vi "AlloysLogger.vi"() -> ()   [LabVIEW 2014]
uses:
  Typedef_FindPortActions.ctl
  Typedef_TeachLabArduinos.ctl
  Typedef_DataLogger_Actions.ctl
  <vilib>/Utility/file.llb/Write To Spreadsheet File (DBL).vi
panel:
  in  "Time Step (ms)":i32=100 min=5 max=5000 step=1
  out "Elapsed Time (s)":dbl format="%.1f"
  out "Temperature (°C)":dbl format="%.1f"
  in  "Filename Header":string="Data"
  in  "Maximum Log Time (s)":dbl=3600.0
  out "Status":enum16{"Logging", "Stopped"}(ring)=enum."Stopped"
  in  "Logging":cluster{"Start":bool, "Stop":bool}
  out "Last Save's Filename":string
  in  "Save Data":bool
  in  "Reset Graph":bool
  out "XY Graph":cluster{dbl[], dbl[]}(graph)
  out "Error Out":errorcluster
  in  "Exit Program":bool
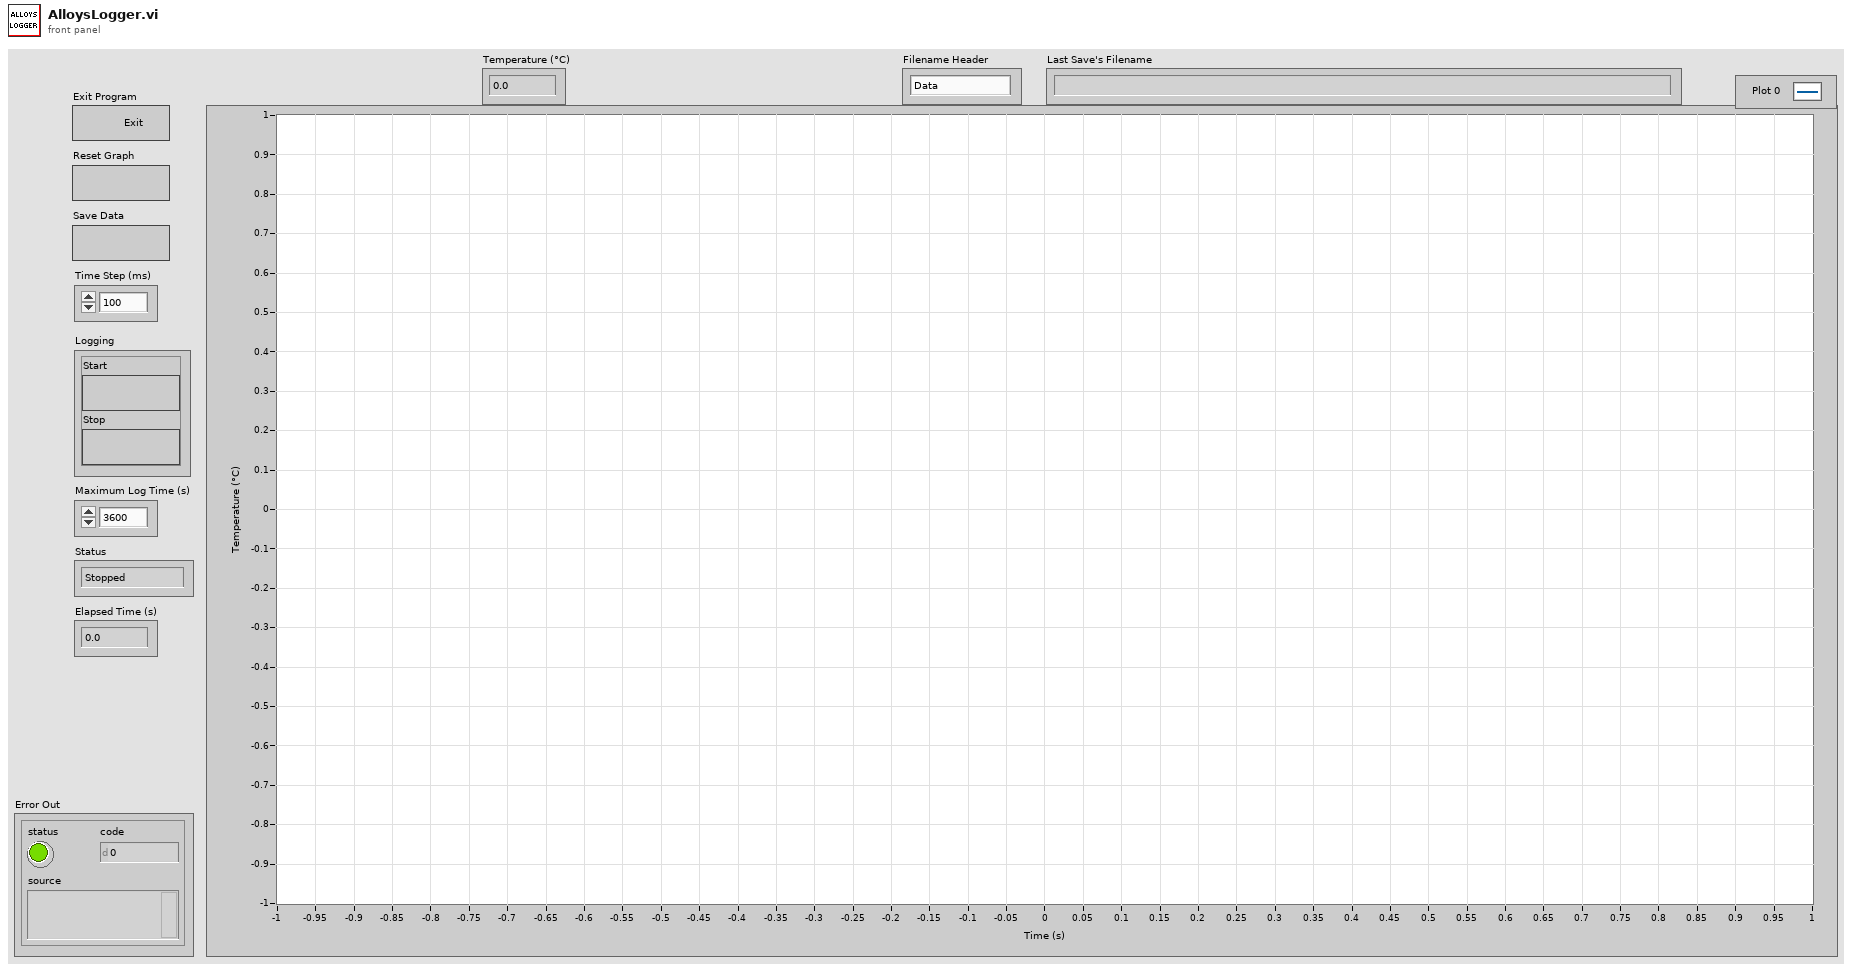
[diagram p1: front panel]
types:
  T1 = typedef "Typedef_FindPortActions.ctl" = enum16{"Reset List", "Find arduinos", "Get COM Port"}
  T2 = typedef "Typedef_TeachLabArduinos.ctl" = enum16{"FH", "AL", "CO"}
  T3 = typedef "Typedef_DataLogger_Actions.ctl" = enum16{"Connect", "Disconnect", "Get Reading", "Set Offset", "Get Offset", "Set Time Step", "Get Time Step", "Save Settings", "Disable Readings", "Enable Readings"}
  T4 = enum32{"invalid app kind", "Development System", "Run Time System", "Student Edition", "Embedded LabVIEW", "Evaluation", "Custom"}
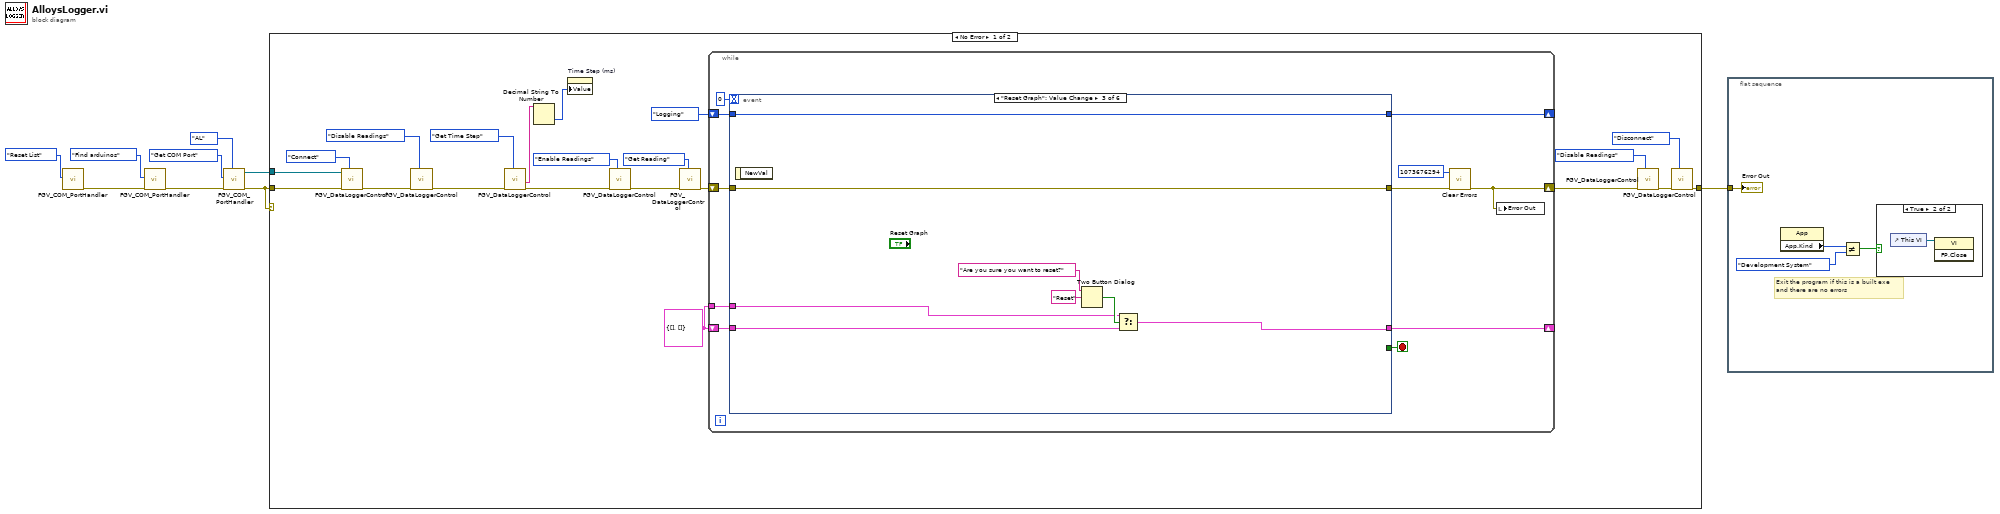
[diagram p0: block diagram]
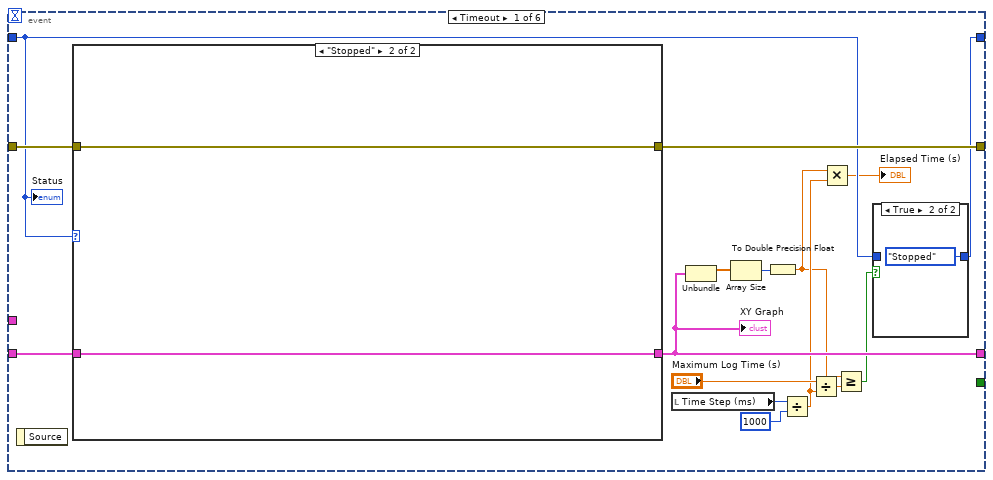
[diagram p3: hidden frame]
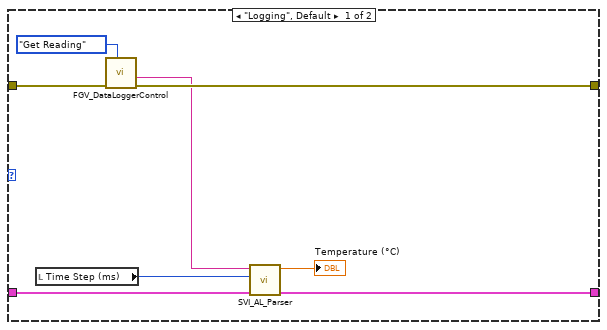
[diagram p5: hidden frame]
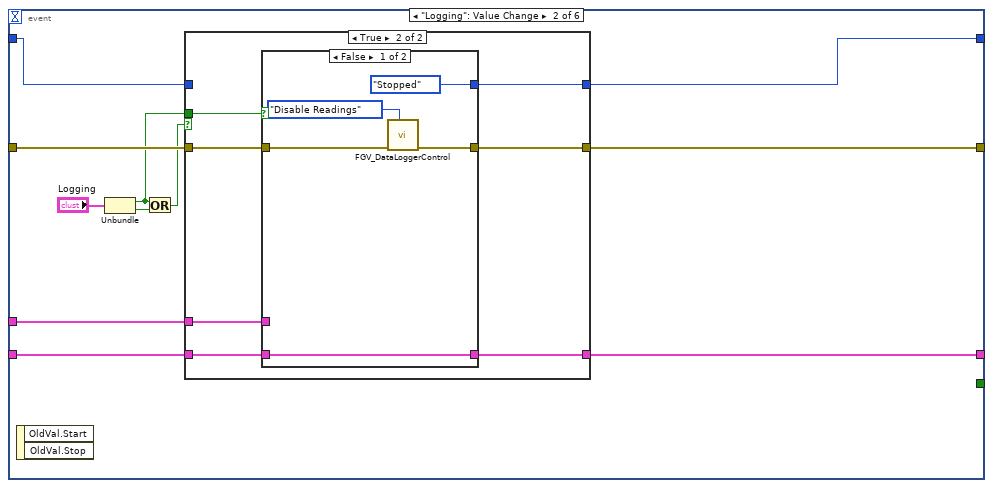
[diagram p6: hidden frame]
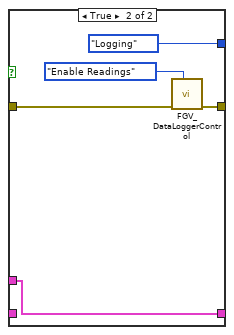
[diagram p8: hidden frame]
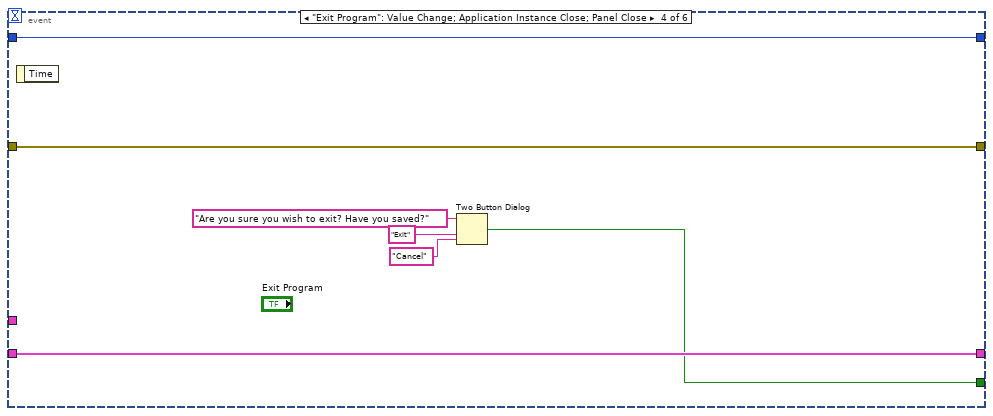
[diagram p9: hidden frame]
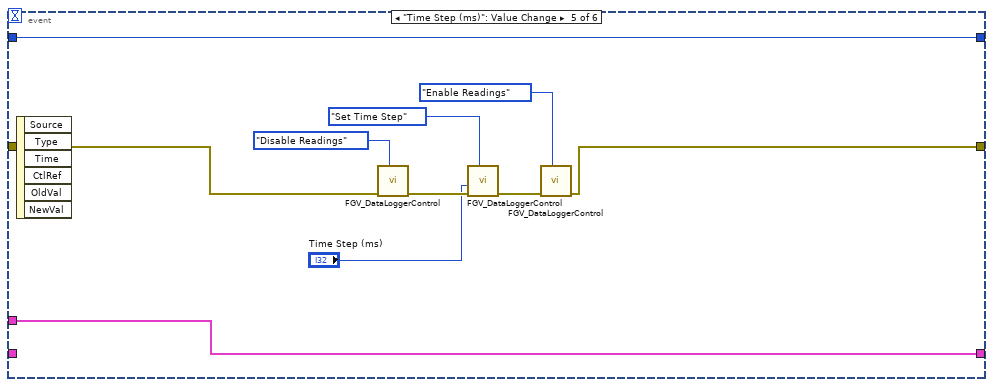
[diagram p10: hidden frame]
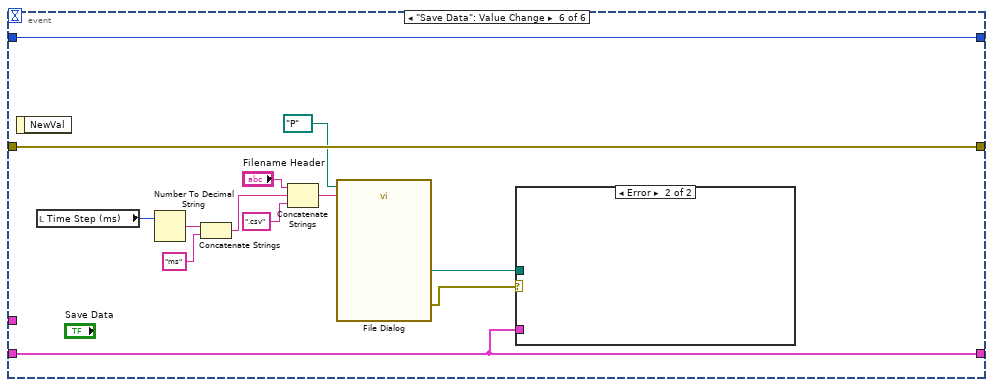
[diagram p11: hidden frame]
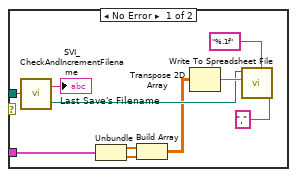
[diagram p12: hidden frame]
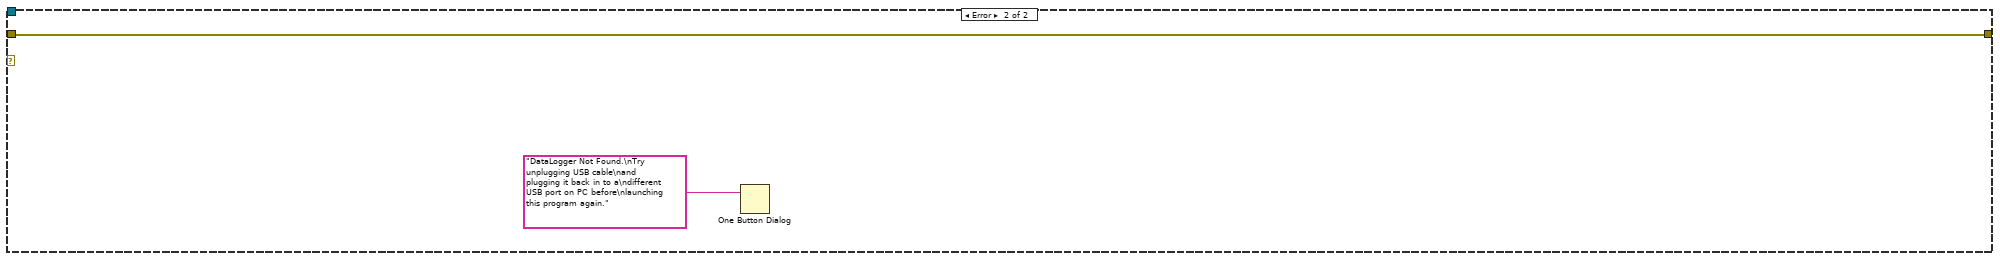
[diagram p13: hidden frame]
diagram:
  n1 = call "FGV_COM_PortHandler.vi"("Action"=Typedef_FindPortActions."Reset List") -> ("Error Out"=w5:errorcluster)  [unwired: 5 in, 2 out]
  n2 = call "FGV_COM_PortHandler.vi"("Error In"=w5, "Action"=Typedef_FindPortActions."Find arduinos") -> ("Error Out"=w9:errorcluster)  [unwired: 4 in, 2 out]
  n3 = call "FGV_COM_PortHandler.vi"("Device"=Typedef_TeachLabArduinos."AL", "Error In"=w9, "Action"=Typedef_FindPortActions."Get COM Port") -> ("Error Out"=w1:errorcluster, "COM Port"=w3:refnum<visa-resource-name>)  [unwired: 3 in, 1 out]
  n4 = case shown="No Error" w1 {
    tunnel: w1 -> [w29 w150]
    tunnel: w3 -> [w28 _]
    tunnel: [w25 w150] -> w2
    frame No Error {
      w14 = cluster{dbl[], dbl[]} {[], []}
      n5 = call "FGV_DataLoggerControl.vi"("Actions"=Typedef_DataLogger_Actions."Connect", "Error In"=w29, "VISA Refnum in"=w28) -> ("Error Out"=w21:errorcluster)  [unwired: 6 in, 2 out]
      n6 = call "FGV_DataLoggerControl.vi"("Actions"=Typedef_DataLogger_Actions."Disable Readings", "Error In"=w21) -> ("Error Out"=w20:errorcluster)  [unwired: 7 in, 2 out]
      n7 = call "FGV_DataLoggerControl.vi"("Actions"=Typedef_DataLogger_Actions."Get Time Step", "Error In"=w20) -> ("Error Out"=w18:errorcluster, "read buffer"=w24:string)  [unwired: 7 in, 1 out]
      n8 = Decimal String To Number(string=w24) -> (number=w23:i32)  [unwired: 2 in, 1 out]
      n9 = property on="Time Step (ms)" class="DigNum (strict)"("Value"=w23) -> ()  [unwired: 2 in, 2 out]
      n10 = call "FGV_DataLoggerControl.vi"("Actions"=Typedef_DataLogger_Actions."Enable Readings", "Error In"=w18) -> ("Error Out"=w10:errorcluster)  [unwired: 7 in, 2 out]
      n11 = call "FGV_DataLoggerControl.vi"("Actions"=Typedef_DataLogger_Actions."Get Reading", "Error In"=w10) -> ("Error Out"=w11:errorcluster)  [unwired: 7 in, 2 out]
      n12 = while {
        shift-right: [w38] -> _
        shift-left: w14 -> [w37]
        tunnel: w14 -> [w36]
        shift-right: [w34] -> _
        shift-left: enum16{"Logging", "Stopped"}."Logging" ("Status") -> [w35]
        shift-right: [w32] -> w16
        shift-left: w11 -> [w41]
        stop <- w40 stop-if-true
        n13 = event shown="[2] \"Reset Graph\": Value Change" {
          selector: _ -> [_ _ _ _ _ _]
          dyn-events: _ -> [_ _ _ _ _ _]
          timeout: 0 -> [_ _ _ _ _ _]
          tunnel: w41 -> [w57 w78 w108 w114 w119 w138]
          tunnel: [w56 w77 w108 w114 w120 w138] -> w31
          tunnel: [_ _ _ w110 _ _] -> w40
          tunnel: [w53 w71 w101 w115 w118 w126] -> w38
          tunnel: w37 -> [w55 w72 w102 w115 _ w126]
          tunnel: w36 -> [_ w70 w103 _ w118 _]
          tunnel: [w46 w80 w107 w109 w117 w130] -> w34
          tunnel: w35 -> [w45 w79 w107 w109 w117 w130]
          event Timeout {
            n14 = event-data() -> ()  [unwired: 1 in, 1 out]
            n15 = case shown="\"Stopped\"" w45 {
              tunnel: w57 -> [w67 w68]
              tunnel: [w66 w68] -> w56
              tunnel: [w63 w69] -> w53
              tunnel: w55 -> [w62 w69]
              frame "Logging", Default {
                n16 = local read "Time Step (ms)"() -> (w60:i32)
                n17 = call "FGV_DataLoggerControl.vi"("Actions"=Typedef_DataLogger_Actions."Get Reading", "Error In"=w67) -> ("Error Out"=w66:errorcluster, "read buffer"=w64:string)  [unwired: 7 in, 1 out]
                n18 = call "SVI_AL_Parser.vi"("Cluster in"=w62, "Time Step (ms)"=w60, "read buffer"=w64) -> ("Cluster out"=w63:cluster{"Array":dbl[], "Array":dbl[]}, "Temperature (°C)"=→"Temperature (°C)":dbl)  [unwired: 3 in]
              }
              frame "Stopped" {
              }
            }
            "XY Graph" <- w53
            n19 = local read "Time Step (ms)"() -> (w52:i32)
            n20 = Unbundle(w53) -> ("Array"=w54:dbl[])  [unwired: 1 out]
            n21 = Array Size(array=w54) -> (size(s)=w48:i32)
            n22 = To Double Precision Float(number=w48) -> (double precision float=w42:dbl)
            n23 = Divide(x=w52, y=1000) -> (x/y=w43:dbl)
            n24 = Divide(x="Maximum Log Time (s)", y=w43) -> (x/y=w49:dbl)
            n25 = Multiply(x=w42, y=w43) -> (x*y=→"Elapsed Time (s)":dbl)
            n26 = Greater Or Equal?(x=w42, y=w49) -> (x >= y?=w47:bool)
            n27 = case shown="True" w47 {
              tunnel: [w58 enum16{"Logging", "Stopped"}."Stopped" ("Status")] -> w46
              tunnel: w45 -> [w58 _]
              frame False {
              }
              frame True {
              }
            }
            "Status" <- w45
          }
          event "Logging": Value Change {
            n28 = event-data() -> ()  [unwired: 1 in, 2 out]
            n29 = Unbundle("Logging") -> ("Start"=w73:bool, "Stop"=w75:bool)
            n30 = Or(x=w73, y=w75) -> (x .or. y?=w74:bool)
            n31 = case shown="True" w74 {
              tunnel: [w83 w90] -> w80
              tunnel: w79 -> [w83 _]
              tunnel: w78 -> [w82 w89]
              tunnel: [w82 w88] -> w77
              tunnel: w73 -> [_ w87]
              tunnel: w72 -> [w81 w86]
              tunnel: [w81 w85] -> w71
              tunnel: w70 -> [_ w84]
              frame False {
              }
              frame True {
                n32 = case shown="False" w87 {
                  tunnel: [enum16{"Logging", "Stopped"}."Stopped" ("Status") enum16{"Logging", "Stopped"}."Logging" ("Status")] -> w90
                  tunnel: w89 -> [w92 w98]
                  tunnel: [w93 w97] -> w88
                  tunnel: w86 -> [w91 _]
                  tunnel: [w91 w96] -> w85
                  tunnel: w84 -> [_ w96]
                  frame False {
                    n33 = call "FGV_DataLoggerControl.vi"("Actions"=Typedef_DataLogger_Actions."Disable Readings", "Error In"=w92) -> ("Error Out"=w93:errorcluster)  [unwired: 7 in, 2 out]
                  }
                  frame True {
                    n34 = call "FGV_DataLoggerControl.vi"("Actions"=Typedef_DataLogger_Actions."Enable Readings", "Error In"=w98) -> ("Error Out"=w97:errorcluster)  [unwired: 7 in, 2 out]
                  }
                }
              }
            }
          }
          event "Reset Graph": Value Change {
            n35 = event-data() -> ()  [unwired: 1 in, 1 out]
            n36 = Two Button Dialog(message="Are you sure you want to reset?", 2:"Reset" ("T button name (\"OK\")")) -> (T button?=w104:bool)  [unwired: 1 in]
            n37 = Select(t=w103, s=w104, f=w102) -> (s? t:f=w101:cluster{dbl[], dbl[]})
          }
          event "Exit Program": Value Change; Application Instance Close; Panel Close {
            n38 = event-data() -> ()  [unwired: 1 in, 1 out]
            n39 = Two Button Dialog(message="Are you sure you wish to exit? Have you saved?", 1:"Cancel" ("F button name (\"Cancel\")"), 2:"Exit" ("T button name (\"OK\")")) -> (T button?=w110:bool)
          }
          event "Time Step (ms)": Value Change {
            n40 = event-data() -> ()  [unwired: 1 in, 6 out]
            n41 = call "FGV_DataLoggerControl.vi"("Actions"=Typedef_DataLogger_Actions."Disable Readings", "Error In"=w119) -> ("Error Out"=w123:errorcluster)  [unwired: 7 in, 2 out]
            n42 = call "FGV_DataLoggerControl.vi"("Actions"=Typedef_DataLogger_Actions."Set Time Step", "Error In"=w123, "Value"="Time Step (ms)") -> ("Error Out"=w121:errorcluster)  [unwired: 6 in, 2 out]
            n43 = call "FGV_DataLoggerControl.vi"("Actions"=Typedef_DataLogger_Actions."Enable Readings", "Error In"=w121) -> ("Error Out"=w120:errorcluster)  [unwired: 7 in, 2 out]
          }
          event "Save Data": Value Change {
            n44 = event-data() -> ()  [unwired: 1 in, 1 out]
            n45 = local read "Time Step (ms)"() -> (w131:i32)
            n46 = Number To Decimal String(number=w131) -> (decimal integer string=w132:string)  [unwired: 1 in]
            n47 = Concatenate Strings(w132, "ms" ("string")) -> (w134:string)
            n48 = Concatenate Strings("Filename Header", w134, ".csv" ("default name")) -> (w136:string)
            n49 = call "File Dialog"("start path"=path "P:/", "default name"=w136) -> ("selected path"=w137:path, "error out"=w128:errorcluster)  [unwired: 10 in, 2 out]
            n50 = case shown="Error" w128 {
              tunnel: w126 -> [w139 _]
              tunnel: w137 -> [w145 _]
              frame No Error {
                n51 = call "SVI_CheckAndIncrementFilename.vi"("selected path"=w145) -> ("Filename"=→"Last Save's Filename":string, "File Path"=w142:path)
                n52 = Unbundle(w139) -> (w147:dbl[], w148:dbl[])
                n53 = Build Array(w147, w148) -> (w141:dbl[][])
                n54 = Transpose 2D Array(2D array=w141) -> (transposed array=w143:dbl[][])
                n55 = call-poly <vilib>:"Write To Spreadsheet File.vi"("delimiter (\\t)"="," ("delimiter (\\t)"), "format (%.3f)"="%.1f", "2D data"=w143, "file path (dialog if empty)"=w142) -> ()  [unwired: 4 in, 1 out]
              }
              frame Error {
              }
            }
          }
        }
        n56 = call <vilib>:"Clear Errors.vi"("error in (no error)"=w31, "specific error code to clear (0: all)"=1073676294) -> ("error out"=w32:errorcluster)  [unwired: 4 in, 1 out]
        n57 = local write "Error Out"(w32) -> ()
      }
      n58 = call "FGV_DataLoggerControl.vi"("Actions"=Typedef_DataLogger_Actions."Disable Readings", "Error In"=w16) -> ("Error Out"=w15:errorcluster)  [unwired: 7 in, 2 out]
      n59 = call "FGV_DataLoggerControl.vi"("Actions"=Typedef_DataLogger_Actions."Disconnect", "Error In"=w15) -> ("Error Out"=w25:errorcluster)  [unwired: 7 in, 2 out]
    }
    frame Error {
      n60 = One Button Dialog(message="DataLogger Not Found.\nTry unplugging USB cable\nand plugging it back in to a\ndifferent USB port on PC before\nlaunching this program again.") -> ()  [unwired: 1 in, 1 out]
    }
  }
  n61 = flat-sequence {
    tunnel: w2 -> [w152]
    frame #0 {
      # "Exit the program if this is a built exe\nand there are no errors"
      n62 = property class="App"() -> ("App.Kind"=w153:T4)  [unwired: 2 in, 2 out]
      n63 = Not Equal?(x=w153, y=T4."Development System" ("Application:Kind 2")) -> (x != y?=w151:bool)
      n64 = case shown="True" w151 {
        frame False {
        }
        frame True {
          n65 = control-ref of="This VI"() -> (w155:refnum<vi>)
          n66 = invoke class="VI" method="FP.Close"(reference=w155) -> ()  [unwired: 2 in, 3 out]
        }
      }
      "Error Out" <- w152
    }
  }
